vi "Oscilloscope Calibration Sub VI (FINAL).vi"(2 "VISA resource name":refnum<visa-resource-name>) -> (1 "error out":errorcluster)   [LabVIEW 2017]
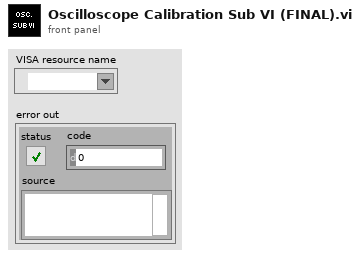
[diagram p1: front panel]
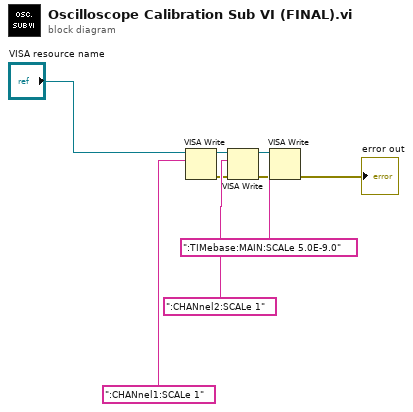
[diagram p0: block diagram]
diagram:
  n1 = VISA Write(VISA resource name="VISA resource name", write buffer=":CHANnel1:SCALe 1") -> (VISA resource name out=w5:refnum<visa-resource-name>, error out=w4:errorcluster)  [unwired: 1 in, 1 out]
  n2 = VISA Write(VISA resource name=w5, write buffer=":CHANnel2:SCALe 1", error in (no error)=w4) -> (VISA resource name out=w6:refnum<visa-resource-name>, error out=w7:errorcluster)  [unwired: 1 out]
  n3 = VISA Write(VISA resource name=w6, write buffer=":TIMebase:MAIN:SCALe 5.0E-9.0", error in (no error)=w7) -> (error out=→"error out":errorcluster)  [unwired: 2 out]
